vi "Configure Thermocouple [TC] Core.vi"(8 "error in (no error)":errorcluster, 9 "ref junc type (Internal)":i32(ring)=1 items=["Internal"=1, "Fixed"=2], 10 "thermocouple type (B)":i32(ring)=1 items=["B"=1, "C"=2, "D"=3, "E"=4, "G"=5, "J"=6, "K"=7, "N"=8, "R"=9, "S"=10, "T"=11, "U"=12, "V"=13], 11 "IVI_DMM in":refnum<class "IVI_DMM.lvclass">) -> (0 "error out":errorcluster, 3 "IVI_DMM out":refnum<class "IVI_DMM.lvclass">)   [LabVIEW 2015, in "IVI_DMM.lvlib" / "IVI_DMM.lvclass"]
doc: "This VI configures the thermocouple type and the reference junction type of the thermocouple for DMMs that take temperature measurements using a thermocouple transducer type.\n\nThis VI affects the behavior of the instrument only if the IviDmm>Temperature Measurements>Transducer Type [TMP] property is set to IVIDMM_VAL_THERMOCOUPLE. \n\nNote:\n\n(1) This VI is part of the IviDmmThermocouple [TC] extension group."
uses:
  IVI_DMM.lvclass
  IVI_DMM.lvclass/IVI_DMM.ctl
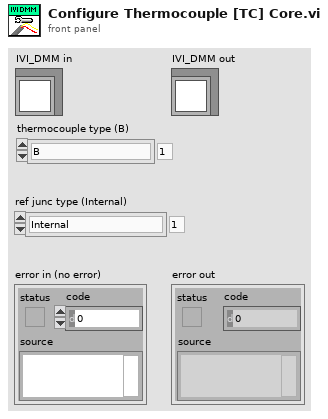
[diagram p1: front panel]
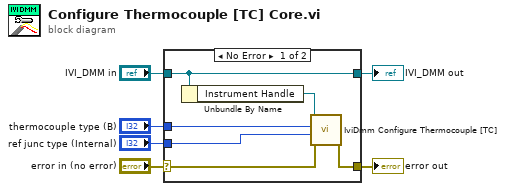
[diagram p0: block diagram]
diagram:
  n1 = case shown="No Error" "error in (no error)" {
    selector: "error in (no error)" -> [w9 w14]
    tunnel: [w11 w14] -> w5
    tunnel: [w12 w13] -> w3
    tunnel: "IVI_DMM in" -> [w12 w13]
    tunnel: "thermocouple type (B)" -> [w8 _]
    tunnel: "ref junc type (Internal)" -> [w7 _]
    frame No Error {
      n2 = Unbundle By Name(w12) -> ("Instrument Handle"=w10:refnum<k15>)
      n3 = call <vilib>:"IviDmm Configure Thermocouple [TC].vi"("error in (no error)"=w9, "ref junc type (Internal)"=w7, "thermocouple type (B)"=w8, "instrument handle"=w10) -> ("error out"=w11:errorcluster)  [unwired: 6 in, 1 out]
    }
    frame Error {
    }
  }
  "error out" <- w5
  "IVI_DMM out" <- w3
